vi "Set Path.vi"(8 "error in (no error)":errorcluster, 10 "File Path":path, 11 "TIFF in":refnum<class "TIFF.lvclass">) -> (0 "error out":errorcluster, 3 "TIFF out":refnum<class "TIFF.lvclass">)   [LabVIEW 2018, in "BinaryTIFF.lvlib" / "TIFF.lvclass"]
uses:
  TIFF.lvclass
  TIFF.lvclass/TIFF.ctl
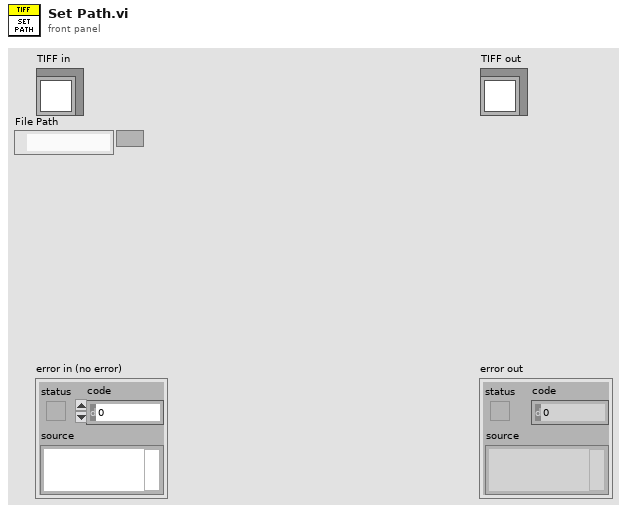
[diagram p1: front panel]
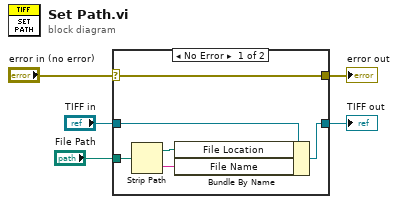
[diagram p0: block diagram]
diagram:
  n1 = case shown="No Error" "error in (no error)" {
    selector: "error in (no error)" -> [w11 w13]
    tunnel: [w11 w13] -> w4
    tunnel: [w6 w12] -> w2
    tunnel: "TIFF in" -> [w10 w12]
    tunnel: "File Path" -> [w7 _]
    frame No Error {
      n2 = Strip Path(path=w7) -> (stripped path=w8:path, name=w9:string)
      n3 = Bundle By Name(cluster=w10, "File Location"=w8, "File Name"=w9) -> (w6:refnum<class "TIFF.lvclass">)
    }
    frame Error {
    }
  }
  "error out" <- w4
  "TIFF out" <- w2
